vi "Digital frequency.vi"() -> ()   [LabVIEW 2018]
uses:
  <vilib>/DAQmx/read.llb/DAQmx Read (Counter 1D DBL 1Chan NSamp).vi
  <vilib>/DAQmx/create/channels.llb/DAQmx Create Channel (CI-Frequency).vi
  <vilib>/DAQmx/configure/timing.llb/DAQmx Timing (Implicit).vi
  <vilib>/DAQmx/miscellaneous.llb/DAQmx Fill In Error Info.vi
  <resource>/objmgr/daqmx.rc
panel:
  out "Waveform Chart 2":dbl[](graph)
  out "data 2":dbl[](array[numeric]) format="%0.2f"
  out "data":dbl[](array[numeric]) format="%0.2f"
  out "Waveform Chart":dbl[](graph)
  in  "stop":bool
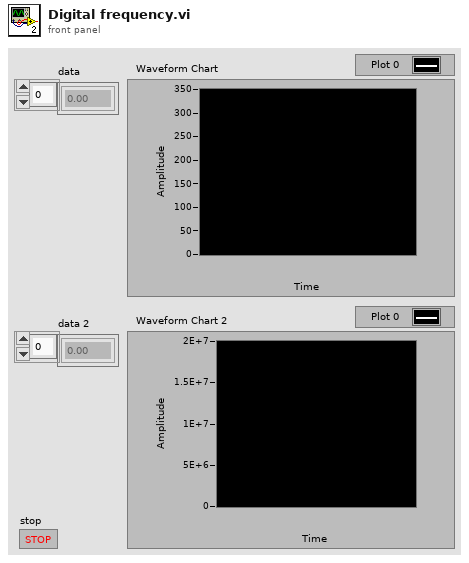
[diagram p1: front panel]
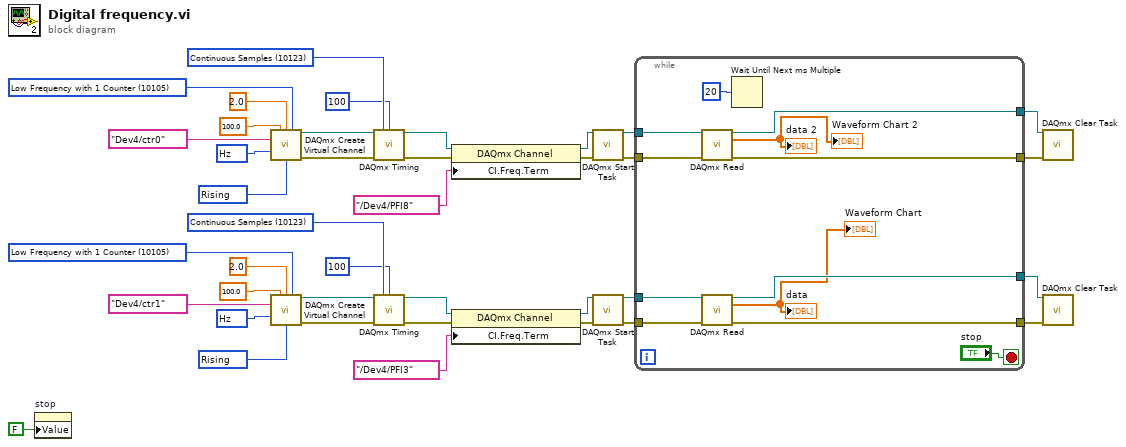
[diagram p0: block diagram]
diagram:
  w10 = 10105 items=["Low Frequency with 1 Counter"=10105, "High Frequency with 2 Counters"=10157, "Large Range with 2 Counters"=10205, "Dynamic Averaging"=16065] ("measurement method")
  w11 = 10280 items=["Rising"=10280, "Falling"=10171] ("starting edge")
  w12 = 10373 items=["Hz"=10373, "Ticks"=10304, "From Custom Scale"=10065] ("units")
  w14 = 10123 items=["Finite Samples"=10178, "Continuous Samples"=10123, "Hardware Timed Single Point"=12522] ("sample mode")
  w26 = 10105 items=["Low Frequency with 1 Counter"=10105, "High Frequency with 2 Counters"=10157, "Large Range with 2 Counters"=10205, "Dynamic Averaging"=16065] ("measurement method")
  w27 = 10280 items=["Rising"=10280, "Falling"=10171] ("starting edge")
  w30 = 10373 items=["Hz"=10373, "Ticks"=10304, "From Custom Scale"=10065] ("units")
  w32 = 10123 items=["Finite Samples"=10178, "Continuous Samples"=10123, "Hardware Timed Single Point"=12522] ("sample mode")
  n1 = property on="stop" class="Bool (strict)"("Value"=FALSE ("stop")) -> ()  [unwired: 2 in, 2 out]
  n2 = call-poly <vilib>:"DAQmx Create Virtual Channel.vi"("maximum value"=100.0, "minimum value"=2.0, "measurement method"=w10, "counter"=tag "Dev4/ctr0", "units"=w12, "starting edge"=w11) -> ("task out"=w15:refnum<k21>, "error out"=w16:errorcluster)  [unwired: 8 in]
  n3 = call-poly <vilib>:"DAQmx Create Virtual Channel.vi"("maximum value"=100.0, "minimum value"=2.0, "measurement method"=w26, "counter"=tag "Dev4/ctr1", "units"=w30, "starting edge"=w27) -> ("task out"=w33:refnum<k21>, "error out"=w34:errorcluster)  [unwired: 8 in]
  n4 = call-poly <vilib>:"DAQmx Timing.vi"("task/channels in"=w15, "sample mode"=w14, "samples per channel"=100, "error in"=w16) -> ("task out"=w9:refnum<k21>, "error out"=w6:errorcluster)  [unwired: 10 in]
  n5 = call-poly <vilib>:"DAQmx Timing.vi"("task/channels in"=w33, "sample mode"=w32, "samples per channel"=100, "error in"=w34) -> ("task out"=w25:refnum<k21>, "error out"=w22:errorcluster)  [unwired: 10 in]
  n6 = property class="DAQmx Channel"(reference=w9, error in=w6, "CI.Freq.Term"=tag "/Dev4/PFI8") -> (reference out=w8:refnum<k21>, error out=w5:errorcluster)
  n7 = property class="DAQmx Channel"(reference=w25, error in=w22, "CI.Freq.Term"=tag "/Dev4/PFI3") -> (reference out=w24:refnum<k21>, error out=w21:errorcluster)
  n8 = call <vilib>:"DAQmx Start Task.vi"("task/channels in"=w8, "error in"=w5) -> ("task out"=w4:refnum<k21>, "error out"=w3:errorcluster)  [unwired: 12 in]
  n9 = call <vilib>:"DAQmx Start Task.vi"("task/channels in"=w24, "error in"=w21) -> ("task out"=w28:refnum<k21>, "error out"=w29:errorcluster)  [unwired: 12 in]
  n10 = while {
    tunnel: [w49] -> w38
    tunnel: w29 -> [w47]
    tunnel: w28 -> [w48]
    tunnel: [w50] -> w39
    tunnel: w4 -> [w43]
    tunnel: w3 -> [w42]
    tunnel: [w41] -> w2
    tunnel: [w40] -> w1
    stop <- "stop" stop-if-true
    n11 = call-poly <vilib>:"DAQmx Read.vi"("task/channels in"=w43, "error in"=w42) -> ("task out"=w41:refnum<k21>, "data"=→"Waveform Chart 2" →"data 2":dbl[], "error out"=w40:errorcluster)  [unwired: 11 in]
    n12 = call-poly <vilib>:"DAQmx Read.vi"("task/channels in"=w48, "error in"=w47) -> ("task out"=w50:refnum<k21>, "data"=→"Waveform Chart" →"data":dbl[], "error out"=w49:errorcluster)  [unwired: 11 in]
    n13 = Wait Until Next ms Multiple(millisecond multiple=u32 20) -> ()  [unwired: 1 out]
  }
  n14 = call <vilib>:"DAQmx Clear Task.vi"("task in"=w2, "error in"=w1) -> ()  [unwired: 13 in, 1 out]
  n15 = call <vilib>:"DAQmx Clear Task.vi"("task in"=w39, "error in"=w38) -> ()  [unwired: 13 in, 1 out]
